vi "Calibration-Line3-CalMain.vi"(8 "error in (no error)":errorcluster, 11 "Calibration-RunTest in":refnum<class "Calibration-RunTest.lvclass">) -> (0 "error out":errorcluster, 3 "Calibration-RunTest out":refnum<class "Calibration-RunTest.lvclass">)   [LabVIEW 2013, in "Calibration-RunTest.lvclass"]
uses:
  Calibration-RunTest.lvclass
  Calibration-RunTest.lvclass/Calibration-RunTest.ctl
  Motion Control/Motion-ControlAll.lvclass
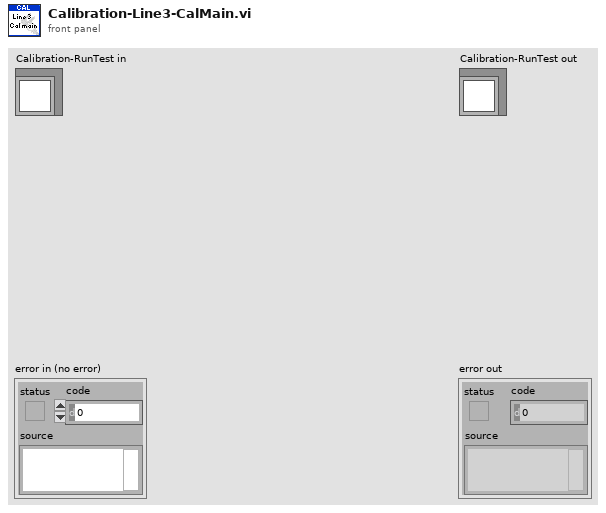
[diagram p1: front panel]
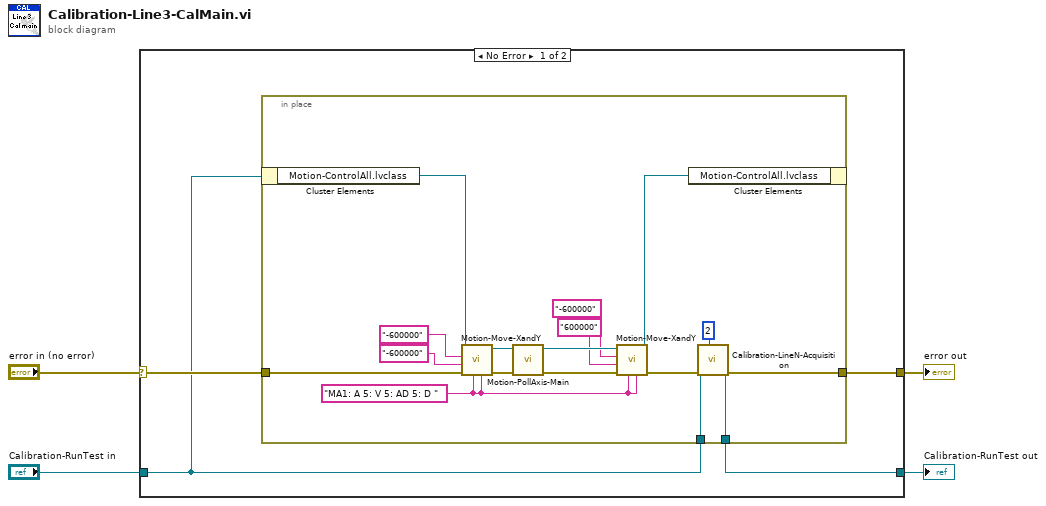
[diagram p0: block diagram]
diagram:
  n1 = case shown="No Error" "error in (no error)" {
    selector: "error in (no error)" -> [w8 w27]
    tunnel: [w7 w27] -> w3
    tunnel: [w5 w26] -> w1
    tunnel: "Calibration-RunTest in" -> [w6 w26]
    frame No Error {
      n2 = in-place {
        in-place-border: w8 -> [w16]
        in-place-border: [w11] -> w7
        in-place-border: w6 -> [w13]
        in-place-border: [w10] -> w5
        w9 = "MA1: A 5: V 5: AD 5: D " ("concatenated string")
        n3 = in-place-cluster #1(w6) -> ("Motion-ControlAll.lvclass"=w17:refnum<class "Motion-ControlAll.lvclass">)
        n4 = call "Motion-Move-XandY.vi"("Y Drive Acc/Speed/Velocity"=w9, "X Drive Acc/Speed/Velocity"=w9, "error in (no error)"=w16, "X Coordinates"="-600000", "Y Coordinates"="-600000", "Motion-ControlAll in"=w17) -> ("error out"=w19:errorcluster, "Motion-ControlAll out"=w18:refnum<class "Motion-ControlAll.lvclass">)  [unwired: 4 in]
        n5 = call "Motion-PollAxis-Main.vi"("error in (no error)"=w19, "Motion-ControlAll in"=w18) -> ("error out"=w24:errorcluster, "Motion-ControlAll out"=w25:refnum<class "Motion-ControlAll.lvclass">)  [unwired: 8 in]
        n6 = call "Motion-Move-XandY.vi"("Y Drive Acc/Speed/Velocity"=w9, "X Drive Acc/Speed/Velocity"=w9, "error in (no error)"=w24, "X Coordinates"="600000", "Y Coordinates"="-600000", "Motion-ControlAll in"=w25) -> ("error out"=w15:errorcluster, "Motion-ControlAll out"=w14:refnum<class "Motion-ControlAll.lvclass">)  [unwired: 4 in]
        n7 = in-place-cluster #1("Motion-ControlAll.lvclass"=w14) -> ()  [unwired: 1 out]
        n8 = call "Calibration-LineN-Acquisition.vi"("Cal Line?"=2, "error in (no error)"=w15, "Calibration-RunTest in"=w13) -> ("error out"=w11:errorcluster, "Calibration-RunTest out"=w10:refnum<class "Calibration-RunTest.lvclass">)  [unwired: 7 in]
      }
    }
    frame Error {
    }
  }
  "error out" <- w3
  "Calibration-RunTest out" <- w1
